vi "Main.vi"() -> ()   [LabVIEW 2019, in "Ex1_server.lvlib" / "Ex1_server.lvclass"]
uses:
  Ex1_server.lvclass
  typeDefs/Server State Data.ctl
  TemperatureSensor/TemperatureSensor.lvclass
panel:
  out "Listening Port":i32
  in  "Stop":bool
  in  "Enable Async Mode":bool
  in  "Server Address":string="localhost:50051"
  in  "Server Certificate File (.crt)":path
  in  "Server Key File (.key)":path
  # "Note: If you want the service to auto find the listening port, then enter the port number in \"Server Address\" as 0. Ex: localhost:0"
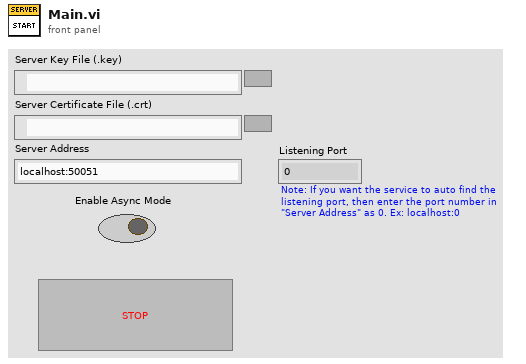
[diagram p1: front panel]
types:
  T1 = typedef "Ex1_server.lvlib/Ex1_server.lvclass/Server State Data.ctl" = cluster{"sensor":refnum<class "TemperatureSensor.lvclass">}
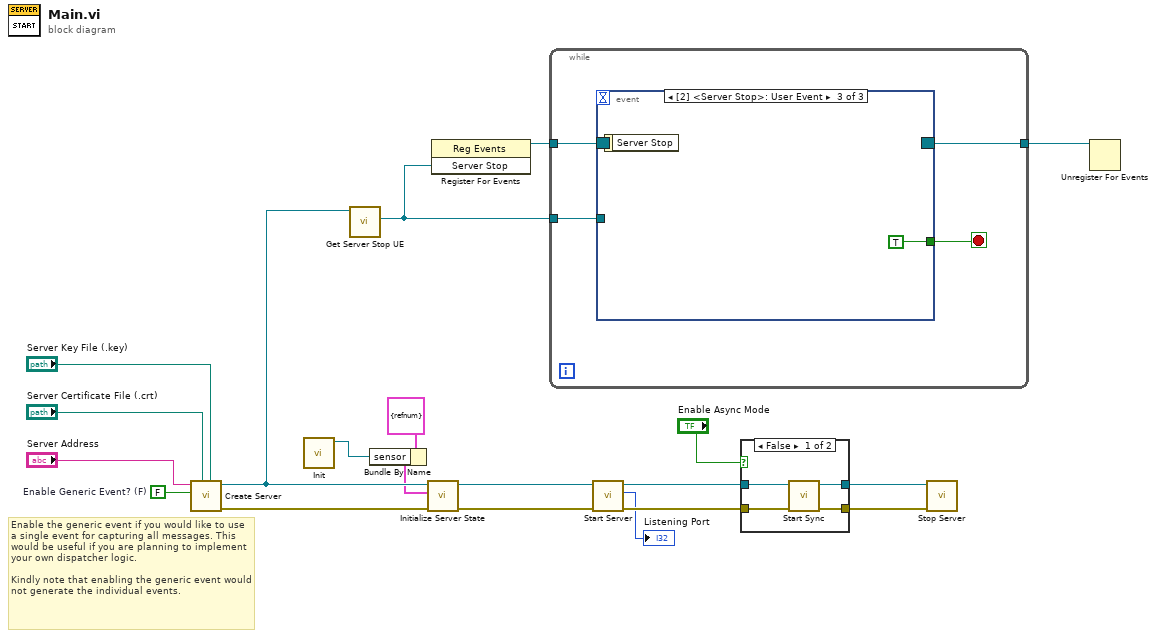
[diagram p0: block diagram]
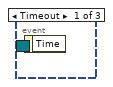
[diagram p2: hidden frame]
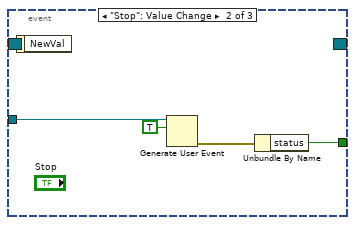
[diagram p3: hidden frame]
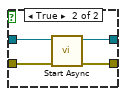
[diagram p4: hidden frame]
diagram:
  w2 = FALSE  # Enable Generic Event? (F)
  # "Enable the generic event if you would like to use a single event for capturing all messages. This would be useful if you are planning to implement your own dispatcher logic. \n\nKindly note that enabling the generic event would not generate the individual events."
  n1 = call "Create Server.vi"("Server Key File (.key)"="Server Key File (.key)", "Server Certificate File (.crt)"="Server Certificate File (.crt)", "Enable Generic Event? (F)"=w2, "Server Address"="Server Address") -> ("error out"=w9:errorcluster, "gRPC Server out"=w6:refnum<class "Ex1_server.lvclass">)  [unwired: 6 in]
  n2 = call "Init.vi"() -> ("TemperatureSensor out"=w1:refnum<class "TemperatureSensor.lvclass">)  [unwired: 10 in, 1 out]
  n3 = call "Get Server Stop UE.vi"("OOP Server in"=w6) -> ("Server Stop"=w10:refnum<user-event>)  [unwired: 9 in, 1 out]
  n4 = Bundle By Name(cluster=T1 {"sensor"=refnum} ("Initial State"), "sensor"=w1) -> (w4:T1)
  n5 = call "Initialize Server State.vi"("error in (no error)"=w9, "Initial State"=w4, "gRPC Server in"=w6) -> ("error out"=w8:errorcluster, "gRPC Server out"=w7:refnum<class "Ex1_server.lvclass">)  [unwired: 7 in]
  n6 = register-events(w10) -> (reference out=w12:refnum<event-registration>)  [unwired: 2 in, 1 out]
  n7 = while {
    tunnel: w10 -> [w24]
    tunnel: w12 -> [w23]
    tunnel: [w21] -> w11
    stop <- w22 stop-if-true
    n8 = event shown="[2] <Server Stop>: User Event" {
      selector: w23 -> [_ _ _]
      dyn-events: [_ _ _] -> w21
      timeout: _ -> [_ _ _]
      tunnel: w24 -> [_ w28 _]
      tunnel: [_ w25 TRUE] -> w22
      event Timeout {
        n9 = event-data() -> ()  [unwired: 1 in, 1 out]
      }
      event "Stop": Value Change {
        n10 = event-data() -> ()  [unwired: 1 in, 1 out]
        n11 = Generate User Event(user event=w28, event data cluster=TRUE ("event data")) -> (error out=w26:errorcluster)  [unwired: 2 in, 1 out]
        n12 = Unbundle By Name(w26) -> ("status"=w25:bool)
      }
      event User Event {
        n13 = event-data() -> ()  [unwired: 1 in, 1 out]
      }
    }
  }
  n14 = call "Start Server.vi"("error in (no error)"=w8, "gRPC Server in"=w7) -> ("error out"=w20:errorcluster, "Listening Port"=→"Listening Port":i32, "gRPC Server out"=w19:refnum<class "Ex1_server.lvclass">)  [unwired: 7 in]
  n15 = case shown="False" "Enable Async Mode" {
    tunnel: w20 -> [w33 w37]
    tunnel: w19 -> [w32 w36]
    tunnel: [w31 w34] -> w18
    tunnel: [w30 w35] -> w17
    frame False {
      n16 = call "Start Sync.vi"("error in (no error)"=w33, "gRPC Server in"=w32) -> ("error out"=w31:errorcluster, "gRPC Server out"=w30:refnum<class "Ex1_server.lvclass">)  [unwired: 8 in]
    }
    frame True {
      n17 = call "Start Async.vi"("error in (no error)"=w37, "gRPC Server in"=w36) -> ("error out"=w34:errorcluster, "gRPC Server out"=w35:refnum<class "Ex1_server.lvclass">)  [unwired: 8 in]
    }
  }
  n18 = call "Stop Server.vi"("error in (no error)"=w18, "gRPC Server in"=w17) -> ()  [unwired: 9 in, 1 out]
  n19 = Unregister For Events(event registration refnum=w11) -> ()  [unwired: 1 in, 1 out]
